vi "finalize digest.vi"(8 "error in":errorcluster, 11 "lvlibcrypto digest in":refnum<class "lvlibcrypto digest.lvclass">) -> (0 "error out":errorcluster, 3 "digest":string)   [LabVIEW 2016, in "lvlibcrypto digest.lvclass"]
uses:
  lvlibcrypto digest.lvclass
  lvlibcrypto digest.lvclass/lvlibcrypto digest.ctl
  lv tls dll.lvlib
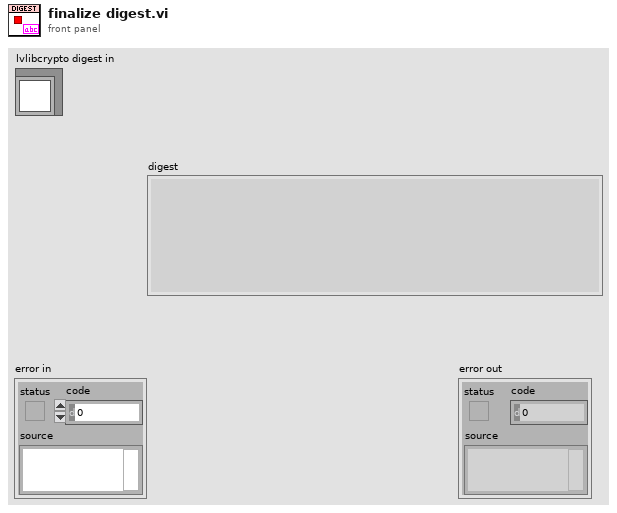
[diagram p1: front panel]
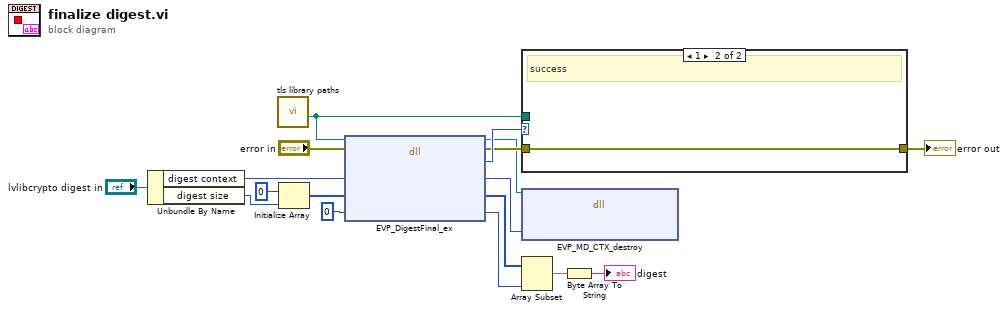
[diagram p0: block diagram]
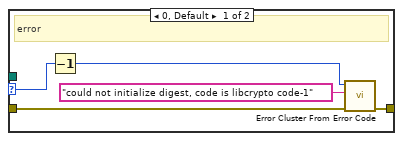
[diagram p2: hidden frame]
diagram:
  n1 = Unbundle By Name("lvlibcrypto digest in") -> ("digest context"=w10:u64, "digest size"=w1:i32)
  n2 = call "tls library paths.vi"() -> ("libcrypto"=w11:path)  [unwired: 8 in, 3 out]
  n3 = Initialize Array(u8 0, w1) -> (w8:u8[])
  n4 = dll-call lib="C:/Users/IEUser/Desktop/tlssimple/libcrypto-41.dll" fn="EVP_DigestFinal_ex"(path in=w11, error in="error in", "context"=w10, "digest"=w8, "length"=u32 0) -> (path out=w13:path, error out=w15:errorcluster, "ret"=w16:i32, "context"=w12:u64, "digest"=w6:u8[], "length"=w5:u32)  [unwired: 1 in]
  n5 = case shown="1" w16 {
    selector: w16 -> [w20 _]
    tunnel: [w21 w23] -> w14
    tunnel: w15 -> [w22 w23]
    tunnel: w11 -> [_ _]
    frame 0, Default {
      # "error"
      n6 = Decrement(x=w20) -> (x-1=w19:i32)
      n7 = call <vilib>:"Error Cluster From Error Code.vi"("error in (no error)"=w22, "error message (\"\")"="could not initialize digest, code is libcrypto code-1" ("error message (\"\")"), "error code (0)"=w19) -> ("error out"=w21:errorcluster)  [unwired: 6 in]
    }
    frame 1 {
      # "success"
    }
  }
  "error out" <- w14
  n8 = dll-call lib="C:/Users/IEUser/Desktop/tlssimple/libcrypto-41.dll" fn="EVP_MD_CTX_destroy"(path in=w13, "context"=w12) -> ()  [unwired: 4 in, 2 out]
  n9 = Array Subset(array=w6, length=w5) -> (w4:u8[])  [unwired: 1 in]
  n10 = Byte Array To String(unsigned byte array=w4) -> (string=→"digest":string)
